vi "evo_irimager_set_pif_framesync_output.vi"() -> ()   [LabVIEW 2017, in "libirimager_direct_binding.lvlib"]
uses:
  libirimager_direct_binding.lvlib
  labview/libirimager.dll
panel:
  in  "AO Output Mode":T1(ring)
  out "Function Return":i32
  in  "Analog Value":sgl=10.0
  in  "AO Channel Id":u32
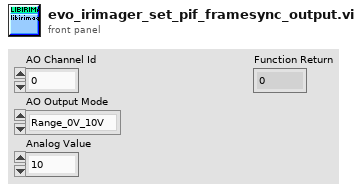
[diagram p1: front panel]
types:
  T1 = enum32{"Range_0V_10V", "Range_0mA_20mA", "Range_4mA_20mA"}
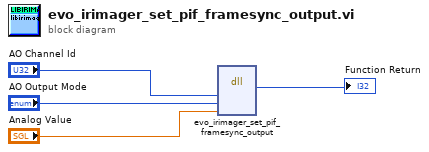
[diagram p0: block diagram]
diagram:
  n1 = dll-call lib="C:/Users/HelmutEngelhardt/Documents/labview/libirimager.dll" fn="evo_irimager_set_pif_framesync_output"("aoChannelId"="AO Channel Id", "analogOutputMode"="AO Output Mode", "analogValue"="Analog Value") -> ("error"=→"Function Return":i32)  [unwired: 6 in, 2 out]
